vi "Save calibration profile - create folder.vi"(8 "error in (no error)":errorcluster) -> (0 "error out":errorcluster, 2 "String":string, 3 "created path":path)   [LabVIEW 2020]
uses:
  Logging/Typedefs/Experiment folder base name.ctl
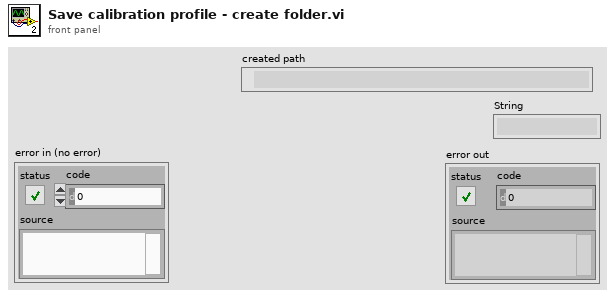
[diagram p1: front panel]
types:
  T1 = typedef "Experiment folder base name.ctl" = enum16{"TimeLapse", "FunctAcq", "ParSweep", "CalibProfl"}
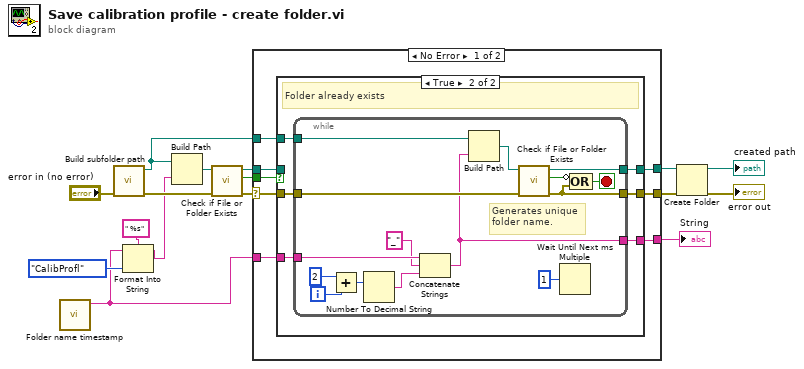
[diagram p0: block diagram]
diagram:
  n1 = call "Folder name timestamp.vi"() -> ("date/time string"=w1:string)  [unwired: 11 in]
  n2 = call "Build subfolder path.vi"("error in (no error)"="error in (no error)") -> ("error out"=w16:errorcluster, "Daily folder or sub-folder path"=w15:path)  [unwired: 9 in]
  n3 = Format Into String(format string=" %s" ("name or relative path"), initial string=w1, Experiment_folder_base_name."CalibProfl" ("Experiment folder base name")) -> (resulting string=w2:string)  [unwired: 1 in, 1 out]
  n4 = Build Path(base path=w15, name or relative path=w2) -> (appended path=w9:path)
  n5 = call <vilib>:"Check if File or Folder Exists.vi"("error in (no error)"=w16, "path"=w9) -> ("error out"=w14:errorcluster, "file or folder exists?"=w10:bool, "dup path"=w11:path)  [unwired: 7 in]
  n6 = case shown="No Error" w14 {
    selector: w14 -> [w18 w51]
    tunnel: w10 -> [w24 _]
    tunnel: w11 -> [w23 w50]
    tunnel: [w22 w50] -> w12
    tunnel: [w21 w51] -> w13
    tunnel: w15 -> [w20 _]
    tunnel: w1 -> [w19 w49]
    tunnel: [w17 w49] -> w5
    frame No Error {
      n7 = case shown="True" w24 {
        tunnel: w23 -> [w27 _]
        tunnel: [w27 w32] -> w22
        tunnel: [w26 w30] -> w21
        tunnel: w20 -> [_ w33]
        tunnel: w19 -> [w25 w31]
        tunnel: w18 -> [w26 w29]
        tunnel: [w25 w28] -> w17
        frame False {
          # "Folder doesn't exist"
        }
        frame True {
          # "Folder already exists"
          n8 = while {
            tunnel: w33 -> [w48]
            tunnel: [w46] -> w32
            tunnel: w31 -> [w38]
            tunnel: [w42] -> w30
            tunnel: w29 -> [w39]
            tunnel: [w37] -> w28
            i -> [w45]
            stop <- w41 stop-if-true
            # "Generates unique\nfolder name."
            n9 = Add(x=2, y=w45) -> (x+y=w35:i32)
            n10 = Number To Decimal String(number=w35) -> (decimal integer string=w34:string)  [unwired: 1 in]
            n11 = Concatenate Strings(w38, "_" ("string"), w34) -> (w37:string)
            n12 = Build Path(base path=w48, name or relative path=w37) -> (appended path=w47:path)
            n13 = call <vilib>:"Check if File or Folder Exists.vi"("error in (no error)"=w39, "path"=w47) -> ("error out"=w42:errorcluster, "file or folder exists?"=w40:bool, "dup path"=w46:path)  [unwired: 7 in]
            n14 = Wait Until Next ms Multiple(millisecond multiple=u32 1) -> ()  [unwired: 1 out]
            n15 = Compound Arithmetic op=OR(invert w40, w42) -> (w41:bool)
          }
        }
      }
    }
    frame Error {
    }
  }
  "String" <- w5
  n16 = Create Folder(path (use dialog)=w12, error in=w13) -> (created path=→"created path":path, error out=→"error out":errorcluster)  [unwired: 1 in, 1 out]
